vi "serpenbot_DDPG_control_parallel.vi"() -> ()   [LabVIEW 2020]
uses:
  <vilib>/Analysis/Matrix/Datatypes/RealMatrix.ctl
  <vilib>/Analysis/Matrix/NI_Matrix.lvlib
  <vilib>/Analysis/NI_AALPro.lvlib
  <vilib>/Analysis/_algsub.llb/Real PseudoInverse Matrix.vi
  <vilib>/Analysis/NI_AALBase.lvlib
  <vilib>/Analysis/baseanly.llb/Real A x B.vi
  <vilib>/Analysis/Matrix/Numeric/Conversions/Array To Matrix - RA.vi
  <vilib>/Analysis/Matrix/Numeric/Subtract/Subtract - RM,RM.vi
panel:
  out "error out Y":errorcluster
  out "error out X":errorcluster
  in  "goal y":dbl
  in  "goal x":dbl
  in  "k":T1
  out "control_loop_time":u32
  in  "stop":bool
  in  "Logging":bool caption="Enable"
  out "current x":dbl
  out "current y":dbl
  out "laser control value":dbl[](array[numeric])
  in  "Diode Current\nSetting":dbl=3.0
  in  "Laser Repetition\nFrequency":i32=50000
  in  "VISA resource name":refnum<visa-resource-name>="COM14"
  in  "baud rate (9600)":u32=9600
  out "error out":errorcluster
  out "Identification system 1":string
  out "Conn. axes system 1":string[](array[string])
  out "Identification system 2":string
  out "Conn. axes system  2":string[](array[string])
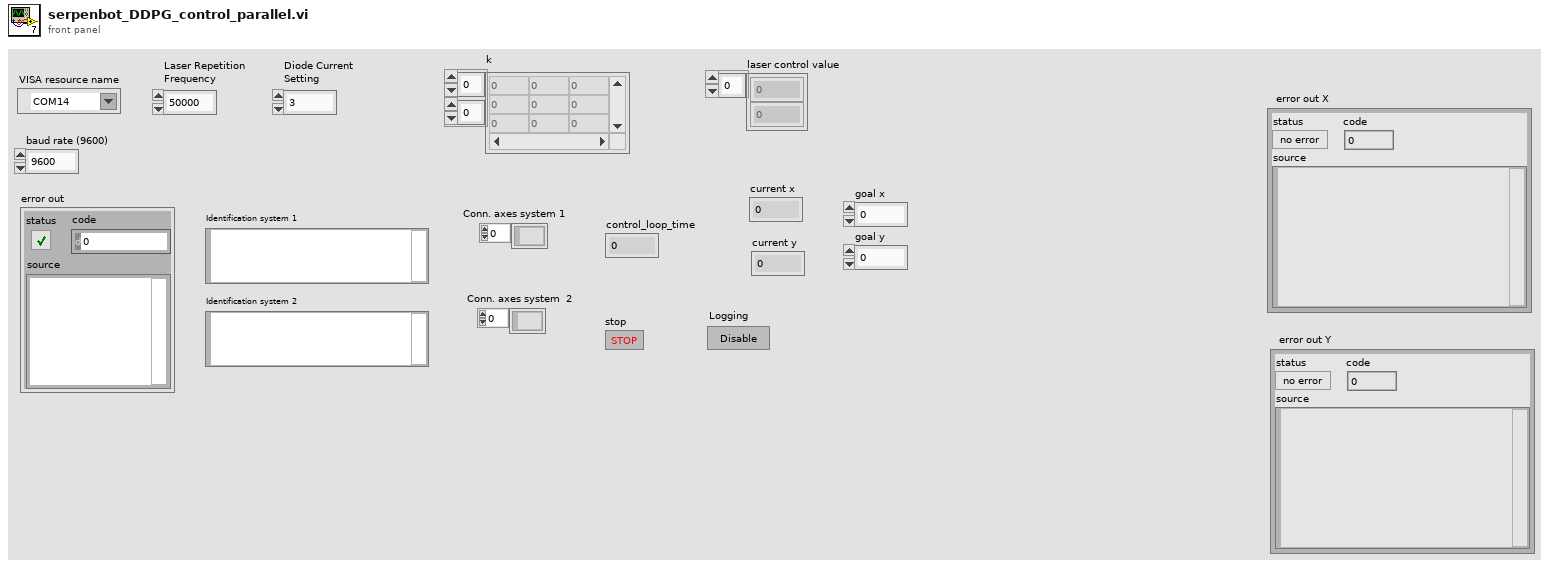
[diagram p1: front panel]
types:
  T1 = typedef "NI_Matrix.lvlib/RealMatrix.ctl" = dbl[][]
  T2 = cluster{"RS232 settings":cluster{"Portnumber":i32, "Baudrate":u16}, "USB settings":cluster{"S/N":string, "USB Search?":bool}, "TCP/IP settings":cluster{"Host address/name":string, "Port":i32, "Board":i32, "TCP/IP Search?":bool}}
  T3 = cluster{"Check FRF?":bool, "Referencing mode":enum16{"FRF (-> FNL)", "FRF", "FNL", "FPL", "RON OFF"}[]}
  T4 = cluster{"Force?":bool, "Dialog?":bool, "Stages":string[]}
  T5 = cluster{"Position":cluster{"x":sgl, "y":sgl}, "Angle":sgl, "Scale":sgl, "Score":sgl, "Bounding Box":cluster{"x":sgl, "y":sgl}[]}[]
  T6 = cluster{"[0]":cluster{"Position":cluster{"x":sgl, "y":sgl}, "Angle":sgl, "Scale":sgl, "Score":sgl, "Bounding Box":cluster{"x":sgl, "y":sgl}[]}, "[1]":cluster{"Position":cluster{"x":sgl, "y":sgl}, "Angle":sgl, "Scale":sgl, "Score":sgl, "Bounding Box":cluster{"x":sgl, "y":sgl}[]}, "[2]":cluster{"Position":cluster{"x":sgl, "y":sgl}, "Angle":sgl, "Scale":sgl, "Score":sgl, "Bounding Box":cluster{"x":sgl, "y":sgl}[]}, "[3]":cluster{"Position":cluster{"x":sgl, "y":sgl}, "Angle":sgl, "Scale":sgl, "Score":sgl, "Bounding Box":cluster{"x":sgl, "y":sgl}[]}, "[4]":cluster{"Position":cluster{"x":sgl, "y":sgl}, "Angle":sgl, "Scale":sgl, "Score":sgl, "Bounding Box":cluster{"x":sgl, "y":sgl}[]}, "[5]":cluster{"Position":cluster{"x":sgl, "y":sgl}, "Angle":sgl, "Scale":sgl, "Score":sgl, "Bounding Box":cluster{"x":sgl, "y":sgl}[]}, "[6]":cluster{"Position":cluster{"x":sgl, "y":sgl}, "Angle":sgl, "Scale":sgl, "Score":sgl, "Bounding Box":cluster{"x":sgl, "y":sgl}[]}, "[7]":cluster{"Position":cluster{"x":sgl, "y":sgl}, "Angle":sgl, "Scale":sgl, "Score":sgl, "Bounding Box":cluster{"x":sgl, "y":sgl}[]}, "[8]":cluster{"Position":cluster{"x":sgl, "y":sgl}, "Angle":sgl, "Scale":sgl, "Score":sgl, "Bounding Box":cluster{"x":sgl, "y":sgl}[]}}
  T7 = cluster{"Position":cluster{"x":sgl, "y":sgl}, "Angle":sgl, "Scale":sgl, "Score":sgl, "Bounding Box":cluster{"x":sgl, "y":sgl}[]}
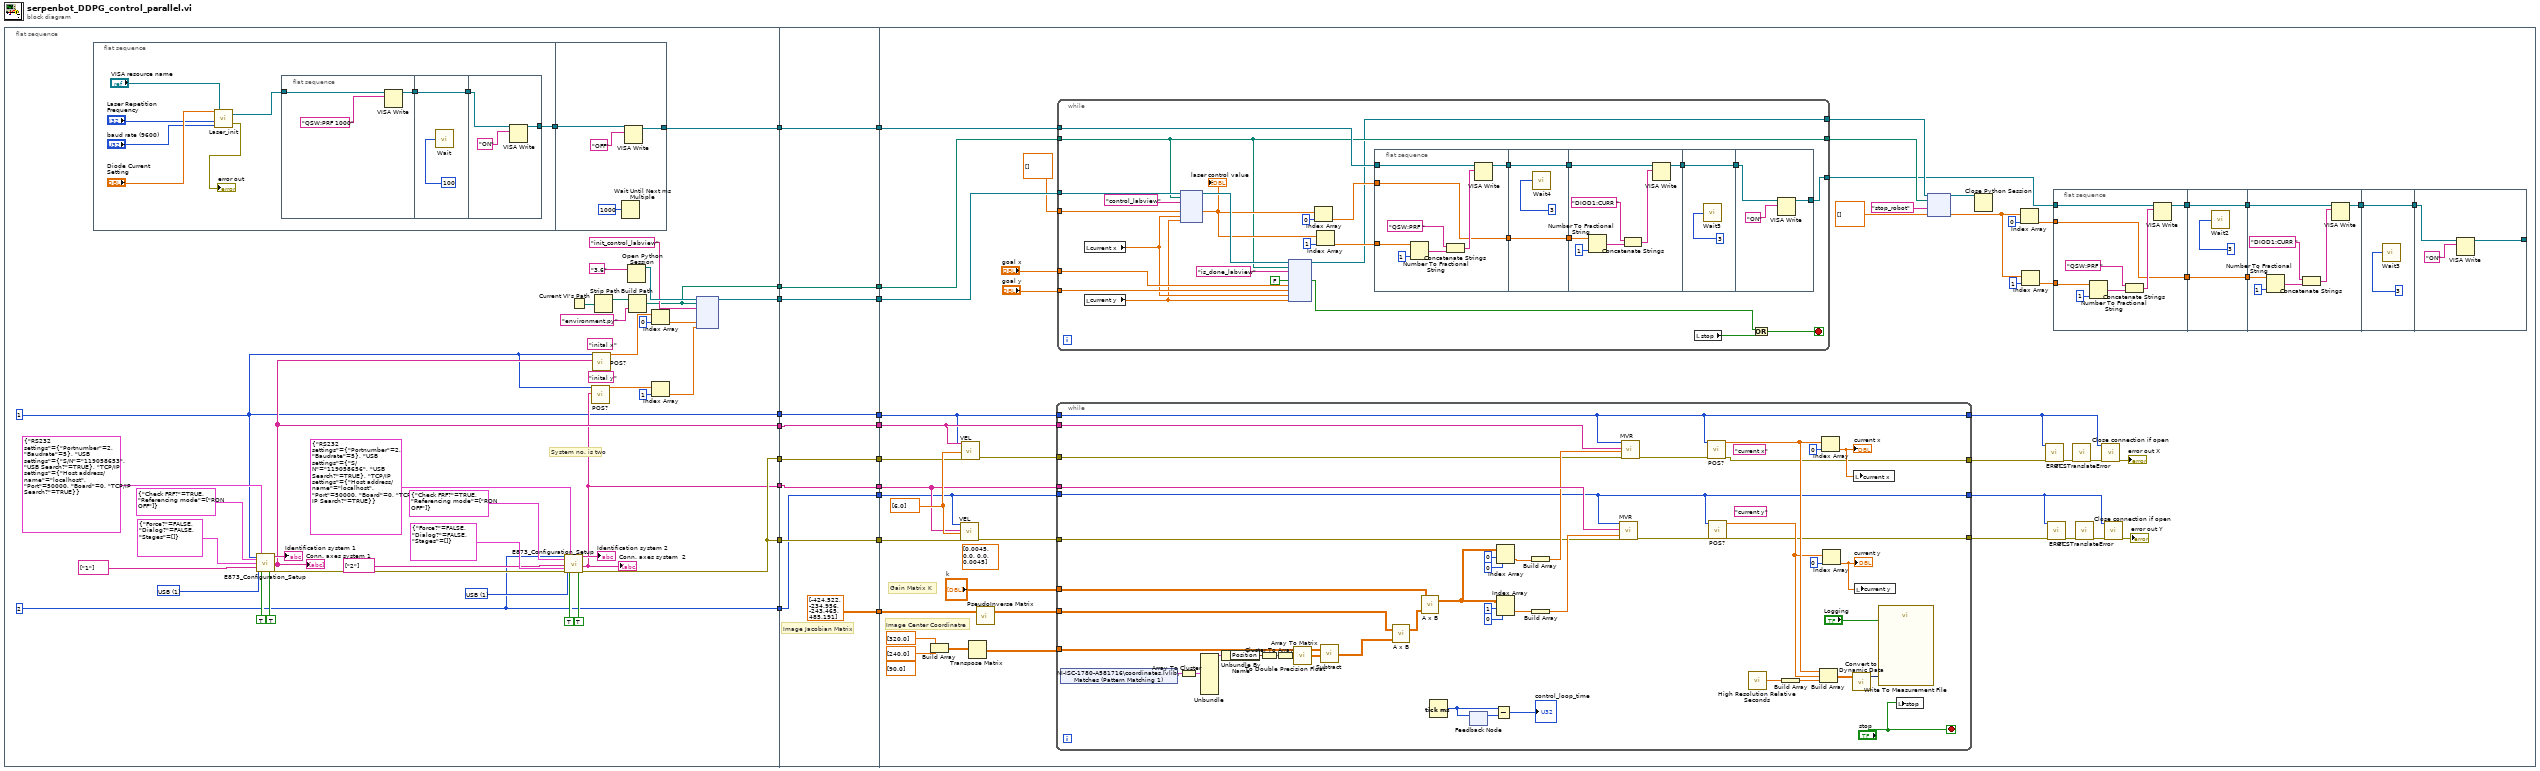
[diagram p0: block diagram]
diagram:
  n1 = flat-sequence {
    tunnel: [w56] -> w19
    tunnel: [w26] -> w18
    tunnel: [w28] -> w17
    tunnel: [w37] -> w16
    tunnel: [w27] -> w15
    tunnel: [w38] -> w14
    tunnel: [w37] -> w13
    tunnel: [w30] -> w12
    tunnel: [w29] -> w11
    tunnel: w19 -> [w88]
    tunnel: [w88] -> w10
    tunnel: w18 -> [w87]
    tunnel: w17 -> [w86]
    tunnel: w16 -> [w85]
    tunnel: w15 -> [w84]
    tunnel: w14 -> [w82]
    tunnel: [w87] -> w9
    tunnel: [w86] -> w8
    tunnel: [w85] -> w7
    tunnel: [w84] -> w6
    tunnel: w13 -> [w83]
    tunnel: [w83] -> w5
    tunnel: [w82] -> w4
    tunnel: [T1 [[-424.522, -234.956], [-243.465, 485.191]] ("J_init 2")] -> w3
    tunnel: w12 -> [w80]
    tunnel: w11 -> [w79]
    tunnel: [w80] -> w2
    tunnel: [w79] -> w1
    tunnel: w10 -> [w105]
    tunnel: w9 -> [w123]
    tunnel: w8 -> [w130]
    tunnel: w7 -> [w133]
    tunnel: w6 -> [w128]
    tunnel: w5 -> [w132]
    tunnel: w4 -> [w122]
    tunnel: w3 -> [w131]
    tunnel: w2 -> [w107]
    tunnel: w1 -> [w106]
    frame #0 {
      (unwired) "inital y"
      (unwired) "inital x"
      w41 = u16 1 items=["RS232", "USB", "TCP/IP"] ("Interface")
      w44 = u16 1 items=["RS232", "USB", "TCP/IP"] ("Interface")
      w38 = 2 ("System no.")
      w26 = 1 ("System no.")
      # "System no. is two"
      n2 = flat-sequence {
        tunnel: [w58] -> w57
        tunnel: w57 -> [w76]
        tunnel: [w75] -> w56
        frame #0 {
          n3 = call "Laser_init.vi"("baud rate (9600)"="baud rate (9600)", "Laser Repetition\nFrequency"="Laser Repetition\nFrequency", "VISA resource name"="VISA resource name", "Diode Current\nSetting"="Diode Current\nSetting") -> ("error out"=→"error out":errorcluster, "VISA Refnum out"=w59:refnum<visa-resource-name>)
          n4 = flat-sequence {
            tunnel: w59 -> [w69]
            tunnel: [w68] -> w66
            tunnel: w66 -> [w71]
            tunnel: [w71] -> w65
            tunnel: w65 -> [w72]
            tunnel: [w73] -> w58
            frame #0 {
              n5 = VISA Write(VISA resource name=w69, write buffer="QSW:PRF 1000" ("string")) -> (VISA resource name out=w68:refnum<visa-resource-name>)  [unwired: 1 in, 2 out]
            }
            frame #1 {
              n6 = call "Wait"("Count(mSec)"=u32 100) -> ()  [unwired: 1 out]
            }
            frame #2 {
              n7 = VISA Write(VISA resource name=w72, write buffer="ON") -> (VISA resource name out=w73:refnum<visa-resource-name>)  [unwired: 1 in, 2 out]
            }
          }
        }
        frame #1 {
          n8 = Wait Until Next ms Multiple(millisecond multiple=u32 1000) -> ()  [unwired: 1 out]
          n9 = VISA Write(VISA resource name=w76, write buffer="OFF") -> (VISA resource name out=w75:refnum<visa-resource-name>)  [unwired: 1 in, 2 out]
        }
      }
      n10 = call "E873_Configuration_Setup.vi"("System no."=w26, "Referencing"=T3 {"Check FRF?"=TRUE, "Referencing mode"=[enum."RON OFF"]}, "Interface"=w44, "All axes?"=TRUE, "Axes to move"=string[] ["1"], "Interface settings"=T2 {"RS232 settings"={"Portnumber"=2, "Baudrate"=5}, "USB settings"={"S/N"="119058653", "USB Search?"=TRUE}, "TCP/IP settings"={"Host address/name"="localhost", "Port"=50000, "Board"=0, "TCP/IP Search?"=TRUE}}, "Stage selection"=T4 {"Force?"=FALSE, "Dialog?"=FALSE, "Stages"=[]}, "Switch servo on?"=TRUE ("Use dialog to define\nconnected stages?")) -> ("Identification"=→"Identification system 1":string, "Conn. \nAxes"=w28:string[], "error out"=w53:errorcluster)  [unwired: 4 in, 5 out]
      "Conn. axes system 1" <- w28
      n11 = call "E873_Configuration_Setup.vi"("System no."=w38, "Referencing"=T3 {"Check FRF?"=TRUE, "Referencing mode"=[enum."RON OFF"]}, "Interface"=w41, "All axes?"=TRUE, "Axes to move"=string[] ["2"], "error in"=w53, "Interface settings"=T2 {"RS232 settings"={"Portnumber"=2, "Baudrate"=5}, "USB settings"={"S/N"="119058656", "USB Search?"=TRUE}, "TCP/IP settings"={"Host address/name"="localhost", "Port"=50000, "Board"=0, "TCP/IP Search?"=TRUE}}, "Stage selection"=T4 {"Force?"=FALSE, "Dialog?"=FALSE, "Stages"=[]}, "Switch servo on?"=TRUE ("Use dialog to define\nconnected stages?")) -> ("Identification"=→"Identification system 2":string, "Conn. \nAxes"=w27:string[], "error out"=w37:errorcluster)  [unwired: 3 in, 5 out]
      "Conn. axes system  2" <- w27
      n12 = Current VI's Path() -> (path=w36:path)
      n13 = call "POS?.vi"("System no."=w26, "Axes to query"=w27) -> ("Position"=w21:dbl[])  [unwired: 3 in, 14 out]
      n14 = call "POS?.vi"("System no."=w26, "Axes to query"=w28) -> ("Position"=w23:dbl[])  [unwired: 3 in, 14 out]
      n15 = Strip Path(path=w36) -> (stripped path=w35:path)  [unwired: 1 out]
      n16 = Open Python Session(python version="3.6" ("Python version")) -> (session out=w32:refnum<k35>)  [unwired: 2 in, 1 out]
      n17 = Build Path(base path=w35, name or relative path="environment.py") -> (appended path=w30:path)
      n18 = Index Array(array=w23, index=0) -> (element=w24:dbl)
      n19 = Index Array(array=w21, index=1) -> (element=w20:dbl)
      n20 = node(w32, w30, "init_control_labview" ("function name"), w24, w20) -> (w29:refnum<k35>)  [unwired: 5 in, 3 out]
    }
    frame #1 {
      # "Image Jacobian Matrix"
    }
    frame #2 {
      w134 = dbl[] [6.0] ("Velocity values")
      (unwired) T1 [[0.0045, 0.0], [0.0, 0.0045]] ("J_init 2")
      (unwired) dbl[] [90.0] ("element")
      # "Gain Matrix K"
      # "Image Center Coordinatre"
      n21 = Build Array(dbl[] [320.0] ("element"), dbl[] [240.0] ("element")) -> (w135:T1)
      n22 = call "VEL.vi"("System no."=w122, "Axes to set"=w128, "Velocity values"=w134, "error in"=w132) -> ("error out"=w127:errorcluster)  [unwired: 2 in, 13 out]
      n23 = call "VEL.vi"("System no."=w123, "Axes to set"=w130, "Velocity values"=w134, "error in"=w133) -> ("error out"=w129:errorcluster)  [unwired: 2 in, 13 out]
      n24 = Transpose Matrix(1:w135) -> (0:w124:T1)
      n25 = call-poly <vilib>:"PseudoInverse Matrix.vi"("Input Matrix"=w131) -> ("PseudoInverse Matrix"=w125:T1)  [unwired: 1 in, 1 out]
      n26 = while {
        tunnel: w127 -> [w216]
        tunnel: w122 -> [w190]
        tunnel: w128 -> [w234]
        tunnel: w129 -> [w217]
        tunnel: w130 -> [w233]
        tunnel: w123 -> [w192]
        tunnel: w125 -> [w222]
        tunnel: "k" -> [w221]
        tunnel: w124 -> [w220]
        tunnel: [w192] -> w91
        tunnel: [w191] -> w92
        tunnel: [w190] -> w90
        tunnel: [w189] -> w89
        stop <- "stop" stop-if-true
        (unwired) "current y"
        (unwired) "current x"
        n27 = shared-variable "NI-ISC-1780-A581716\\coordinates.lvlib\\Matches (Pattern Matching 1)"() -> (w209:T5)  [unwired: 1 in, 1 out]
        n28 = Array To Cluster(array=w209) -> (cluster=w210:T6)
        n29 = Unbundle(w210) -> ("[0]"=w211:T7)  [unwired: 8 out]
        n30 = Unbundle By Name(w211) -> ("Position"=w212:cluster{"x":sgl, "y":sgl})
        n31 = Cluster To Array(cluster=w212) -> (array=w213:sgl[])
        n32 = To Double Precision Float(number=w213) -> (double precision float=w214:dbl[])
        n33 = call-poly <vilib>:"Array To Matrix.vi"("Real 1D Array"=w214) -> ("Real Matrix (Column Vector)"=w208:T1)
        n34 = call-poly <vilib>:"Subtract.vi"("Real Matrix B"=w208, "Real Matrix A"=w220) -> ("A - B"=w228:T1)
        n35 = call-poly <vilib>:"A x B.vi"("B"=w228, "A"=w222) -> ("A x B"=w226:T1)  [unwired: 1 out]
        n36 = call-poly <vilib>:"A x B.vi"("B"=w226, "A"=w221) -> ("A x B"=w227:T1)  [unwired: 1 out]
        n37 = Tick Count (ms)() -> (millisecond timer value=w200:u32)
        n38 = feedback #1() -> (w223:u32)  [unwired: 1 in]
        n39 = feedback-in #1(w200) -> ()
        n40 = Subtract(x=w200, y=w223) -> (x-y=→"control_loop_time":u32)
        n41 = Index Array(array=w227, index (row)=0, index (col)=0) -> (element=w219:dbl)
        n42 = Index Array(array=w227, index (row)=1, index (col)=0) -> (element=w218:dbl)
        n43 = Build Array(w219) -> (w225:dbl[])
        n44 = Build Array(w218) -> (w224:dbl[])
        n45 = call "MVR.vi"("System no."=w190, "Axes to move"=w234, "Position values"=w224, "error in"=w216) -> ("error out"=w201:errorcluster)  [unwired: 1 in, 14 out]
        n46 = call "MVR.vi"("System no."=w192, "Axes to move"=w233, "Position values"=w225, "error in"=w217) -> ("error out"=w202:errorcluster)  [unwired: 1 in, 14 out]
        n47 = call "POS?.vi"("System no."=w192, "error in"=w202) -> ("Position"=w199:dbl[], "error out"=w191:errorcluster)  [unwired: 3 in, 13 out]
        n48 = call "POS?.vi"("System no."=w190, "error in"=w201) -> ("Position"=w197:dbl[], "error out"=w189:errorcluster)  [unwired: 3 in, 13 out]
        n49 = call <vilib>:"High Resolution Relative Seconds.vi"() -> ("relative seconds"=w204:dbl)
        n50 = Build Array(w204) -> (w203:dbl[])
        n51 = Build Array(w199, w197, w203) -> (w206:dbl[][])
        n52 = Index Array(array=w199, index=0) -> (element=w195:dbl)
        "current x" <- w195
        n53 = Index Array(array=w197, index=0) -> (element=w194:dbl)
        "current y" <- w194
        n54 = call "Convert to Dynamic Data"("2D Array"=w206) -> ("Dynamic Data Type"=w205:dynamicdata)  [unwired: 3 in]
        n55 = local write "current x"(w195) -> ()
        n56 = local write "current y"(w194) -> ()
        n57 = call "Write To Measurement File"("Signals"=w205, "Enable"="Logging") -> ()  [unwired: 15 in, 3 out]
        n58 = local write "stop"("stop") -> ()
      }
      n59 = while {
        tunnel: dbl[] [] -> [w150]
        tunnel: "goal x" -> [w149]
        tunnel: "goal y" -> [w148]
        tunnel: w107 -> [w145]
        tunnel: w106 -> [w147]
        tunnel: w105 -> [w146]
        tunnel: [w145] -> w104
        tunnel: [w144] -> w103
        tunnel: [w141] -> w102
        stop <- w142 stop-if-true
        n60 = local read "current x"() -> (w140:dbl)
        n61 = local read "current y"() -> (w139:dbl)
        n62 = node(w147, w145, "control_labview" ("function name"), w150, w140, w139) -> (w158:refnum<k35>, w152:dbl[])  [unwired: 3 in, 3 out]
        "laser control value" <- w152
        n63 = node(w158, w145, "is_done_labview" ("function name"), FALSE, w149, w148, w140, w139) -> (w144:refnum<k35>, w138:bool)  [unwired: 5 in, 3 out]
        n64 = Index Array(array=w152, index=0) -> (element=w155:dbl)
        n65 = Index Array(array=w152, index=1) -> (element=w151:dbl)
        n66 = flat-sequence {
          tunnel: w146 -> [w169]
          tunnel: [w168] -> w165
          tunnel: w151 -> [w167]
          tunnel: w155 -> [w166]
          tunnel: [w166] -> w164
          tunnel: [w176] -> w163
          tunnel: [w174] -> w162
          tunnel: w165 -> [w176]
          tunnel: w164 -> [w174]
          tunnel: [w183] -> w161
          tunnel: w163 -> [w181]
          tunnel: w162 -> [w178]
          tunnel: w161 -> [w185]
          tunnel: [w185] -> w160
          tunnel: w160 -> [w187]
          tunnel: [w186] -> w141
          frame #0 {
            n67 = Number To Fractional String(number=w167, precision (6)=i16 1) -> (F-format string=w172:string)  [unwired: 2 in]
            n68 = Concatenate Strings("QSW:PRF " ("string"), w172) -> (w173:string)
            n69 = VISA Write(VISA resource name=w169, write buffer=w173) -> (VISA resource name out=w168:refnum<visa-resource-name>)  [unwired: 1 in, 2 out]
          }
          frame #1 {
            n70 = call "Wait4"("Count(mSec)"=u32 3) -> ()  [unwired: 1 out]
          }
          frame #2 {
            n71 = Number To Fractional String(number=w178, precision (6)=i16 1) -> (F-format string=w179:string)  [unwired: 2 in]
            n72 = Concatenate Strings("DIOD1:CURR " ("string"), w179) -> (w182:string)
            n73 = VISA Write(VISA resource name=w181, write buffer=w182) -> (VISA resource name out=w183:refnum<visa-resource-name>)  [unwired: 1 in, 2 out]
          }
          frame #3 {
            n74 = call "Wait5"("Count(mSec)"=u32 3) -> ()  [unwired: 1 out]
          }
          frame #4 {
            n75 = VISA Write(VISA resource name=w187, write buffer="ON") -> (VISA resource name out=w186:refnum<visa-resource-name>)  [unwired: 1 in, 2 out]
          }
        }
        n76 = local read "stop"() -> (w143:bool)
        n77 = Or(x=w138, y=w143) -> (x .or. y?=w142:bool)
      }
      n78 = node(w103, w104, "stop_robot" ("function name"), dbl[] []) -> (w113:refnum<k35>, w108:dbl[])  [unwired: 1 in, 3 out]
      n79 = Close Python Session(session in=w113) -> ()  [unwired: 1 in, 1 out]
      n80 = Index Array(array=w108, index=0) -> (element=w110:dbl)
      n81 = Index Array(array=w108, index=1) -> (element=w109:dbl)
      n82 = call "ERR?.vi"("System no."=w91, "error in"=w92) -> ("error out"=w96:errorcluster)  [unwired: 17 out]
      n83 = call "ERR?.vi"("System no."=w90, "error in"=w89) -> ("error out"=w93:errorcluster)  [unwired: 17 out]
      n84 = flat-sequence {
        tunnel: w102 -> [w238]
        tunnel: [w237] -> w121
        tunnel: w109 -> [w236]
        tunnel: w110 -> [w235]
        tunnel: [w235] -> w120
        tunnel: [w245] -> w119
        tunnel: [w243] -> w118
        tunnel: w121 -> [w245]
        tunnel: w120 -> [w243]
        tunnel: [w252] -> w117
        tunnel: w119 -> [w250]
        tunnel: w118 -> [w247]
        tunnel: w117 -> [w254]
        tunnel: [w254] -> w116
        tunnel: w116 -> [w256]
        tunnel: [w255] -> _
        frame #0 {
          n85 = Number To Fractional String(number=w236, precision (6)=i16 1) -> (F-format string=w241:string)  [unwired: 2 in]
          n86 = Concatenate Strings("QSW:PRF " ("string"), w241) -> (w242:string)
          n87 = VISA Write(VISA resource name=w238, write buffer=w242) -> (VISA resource name out=w237:refnum<visa-resource-name>)  [unwired: 1 in, 2 out]
        }
        frame #1 {
          n88 = call "Wait2"("Count(mSec)"=u32 3) -> ()  [unwired: 1 out]
        }
        frame #2 {
          n89 = Number To Fractional String(number=w247, precision (6)=i16 1) -> (F-format string=w248:string)  [unwired: 2 in]
          n90 = Concatenate Strings("DIOD1:CURR " ("string"), w248) -> (w251:string)
          n91 = VISA Write(VISA resource name=w250, write buffer=w251) -> (VISA resource name out=w252:refnum<visa-resource-name>)  [unwired: 1 in, 2 out]
        }
        frame #3 {
          n92 = call "Wait3"("Count(mSec)"=u32 3) -> ()  [unwired: 1 out]
        }
        frame #4 {
          n93 = VISA Write(VISA resource name=w256, write buffer="ON") -> (VISA resource name out=w255:refnum<visa-resource-name>)  [unwired: 1 in, 2 out]
        }
      }
      n94 = call "GCSTranslateError.vi"("error in"=w96) -> ("error out"=w97:errorcluster)  [unwired: 18 out]
      n95 = call "GCSTranslateError.vi"("error in"=w93) -> ("error out"=w94:errorcluster)  [unwired: 18 out]
      n96 = call "Close connection if open.vi"("System no."=w91, "error in"=w97) -> ("error out"=→"error out X":errorcluster)  [unwired: 1 in, 16 out]
      n97 = call "Close connection if open.vi"("System no."=w90, "error in"=w94) -> ("error out"=→"error out Y":errorcluster)  [unwired: 1 in, 16 out]
    }
  }
